vi "CreateCommands.vi"   [LabVIEW 2011]
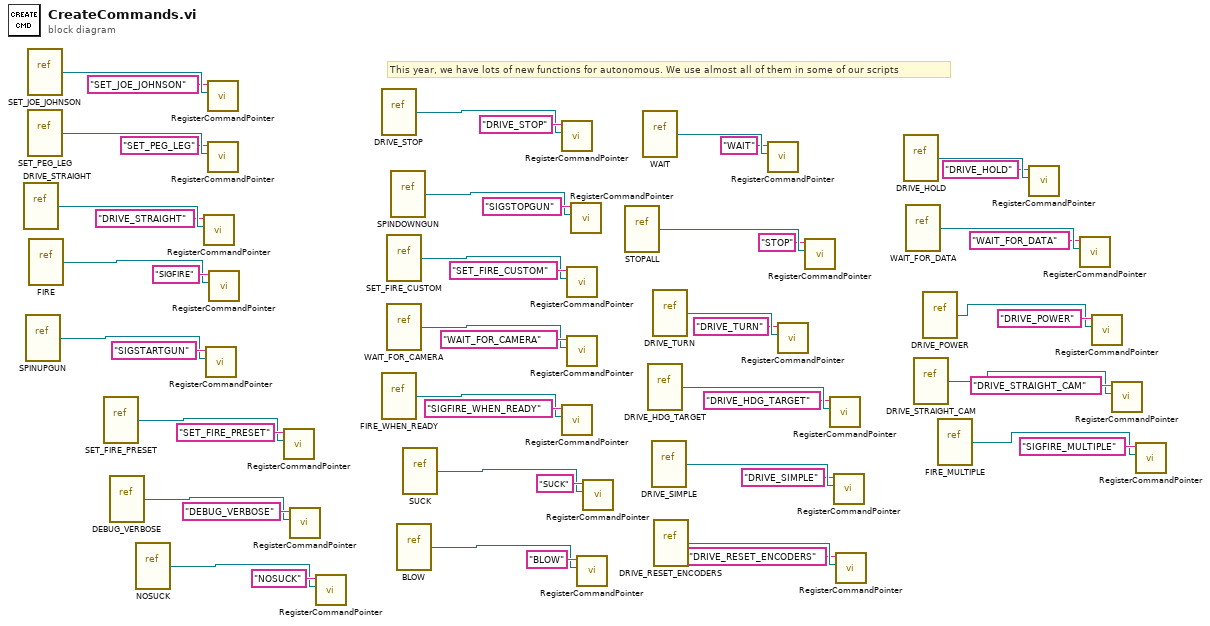
[diagram p0: block diagram]
diagram:
  # "This year, we have lots of new functions for autonomous. We use almost all of them in some of our scripts"
  n1 = vi-ref "DRIVE_STRAIGHT.vi"() -> (w44:refnum<vi>)
  n2 = vi-ref "SPINUPGUN.vi"() -> (w39:refnum<vi>)
  n3 = vi-ref "SET_JOE_JOHNSON.vi"() -> (w48:refnum<vi>)
  n4 = vi-ref "SET_PEG_LEG.vi"() -> (w46:refnum<vi>)
  n5 = vi-ref "FIRE.vi"() -> (w41:refnum<vi>)
  n6 = vi-ref "SET_FIRE_PRESET.vi"() -> (w37:refnum<vi>)
  n7 = vi-ref "DEBUG_VERBOSE.vi"() -> (w35:refnum<vi>)
  n8 = vi-ref "NOSUCK.vi"() -> (w33:refnum<vi>)
  n9 = call "RegisterCommandPointer.vi"("Strict-Typed VI Refnum"=w44, "Name"="DRIVE_STRAIGHT") -> ()  [unwired: 10 out]
  n10 = call "RegisterCommandPointer.vi"("Strict-Typed VI Refnum"=w39, "Name"="SIGSTARTGUN") -> ()  [unwired: 10 out]
  n11 = call "RegisterCommandPointer.vi"("Strict-Typed VI Refnum"=w48, "Name"="SET_JOE_JOHNSON") -> ()  [unwired: 10 out]
  n12 = call "RegisterCommandPointer.vi"("Strict-Typed VI Refnum"=w46, "Name"="SET_PEG_LEG") -> ()  [unwired: 10 out]
  n13 = call "RegisterCommandPointer.vi"("Strict-Typed VI Refnum"=w41, "Name"="SIGFIRE") -> ()  [unwired: 10 out]
  n14 = call "RegisterCommandPointer.vi"("Strict-Typed VI Refnum"=w37, "Name"="SET_FIRE_PRESET") -> ()  [unwired: 10 out]
  n15 = call "RegisterCommandPointer.vi"("Strict-Typed VI Refnum"=w35, "Name"="DEBUG_VERBOSE") -> ()  [unwired: 10 out]
  n16 = call "RegisterCommandPointer.vi"("Strict-Typed VI Refnum"=w33, "Name"="NOSUCK") -> ()  [unwired: 10 out]
  n17 = vi-ref "DRIVE_STOP.vi"() -> (w19:refnum<vi>)
  n18 = vi-ref "FIRE_WHEN_READY.vi"() -> (w27:refnum<vi>)
  n19 = vi-ref "SET_FIRE_CUSTOM.vi"() -> (w23:refnum<vi>)
  n20 = vi-ref "WAIT_FOR_CAMERA.vi"() -> (w25:refnum<vi>)
  n21 = vi-ref "SPINDOWNGUN.vi"() -> (w21:refnum<vi>)
  n22 = vi-ref "BLOW.vi"() -> (w31:refnum<vi>)
  n23 = vi-ref "SUCK.vi"() -> (w29:refnum<vi>)
  n24 = call "RegisterCommandPointer.vi"("Strict-Typed VI Refnum"=w19, "Name"="DRIVE_STOP") -> ()  [unwired: 10 out]
  n25 = call "RegisterCommandPointer.vi"("Strict-Typed VI Refnum"=w27, "Name"="SIGFIRE_WHEN_READY") -> ()  [unwired: 10 out]
  n26 = call "RegisterCommandPointer.vi"("Strict-Typed VI Refnum"=w23, "Name"="SET_FIRE_CUSTOM") -> ()  [unwired: 10 out]
  n27 = call "RegisterCommandPointer.vi"("Strict-Typed VI Refnum"=w25, "Name"="WAIT_FOR_CAMERA") -> ()  [unwired: 10 out]
  n28 = call "RegisterCommandPointer.vi"("Strict-Typed VI Refnum"=w21, "Name"="SIGSTOPGUN") -> ()  [unwired: 10 out]
  n29 = call "RegisterCommandPointer.vi"("Strict-Typed VI Refnum"=w31, "Name"="BLOW") -> ()  [unwired: 10 out]
  n30 = call "RegisterCommandPointer.vi"("Strict-Typed VI Refnum"=w29, "Name"="SUCK") -> ()  [unwired: 10 out]
  n31 = vi-ref "STOPALL.vi"() -> (w52:refnum<vi>)
  n32 = vi-ref "WAIT.vi"() -> (w50:refnum<vi>)
  n33 = vi-ref "DRIVE_HDG_TARGET.vi"() -> (w16:refnum<vi>)
  n34 = vi-ref "DRIVE_SIMPLE.vi"() -> (w14:refnum<vi>)
  n35 = vi-ref "DRIVE_TURN.vi"() -> (w18:refnum<vi>)
  n36 = vi-ref "DRIVE_RESET_ENCODERS.vi"() -> (w12:refnum<vi>)
  n37 = call "RegisterCommandPointer.vi"("Strict-Typed VI Refnum"=w50, "Name"="WAIT") -> ()  [unwired: 10 out]
  n38 = call "RegisterCommandPointer.vi"("Strict-Typed VI Refnum"=w18, "Name"="DRIVE_TURN") -> ()  [unwired: 10 out]
  n39 = call "RegisterCommandPointer.vi"("Strict-Typed VI Refnum"=w52, "Name"="STOP") -> ()  [unwired: 10 out]
  n40 = call "RegisterCommandPointer.vi"("Strict-Typed VI Refnum"=w16, "Name"="DRIVE_HDG_TARGET") -> ()  [unwired: 10 out]
  n41 = call "RegisterCommandPointer.vi"("Strict-Typed VI Refnum"=w14, "Name"="DRIVE_SIMPLE") -> ()  [unwired: 10 out]
  n42 = call "RegisterCommandPointer.vi"("Strict-Typed VI Refnum"=w12, "Name"="DRIVE_RESET_ENCODERS") -> ()  [unwired: 10 out]
  n43 = vi-ref "DRIVE_HOLD.vi"() -> (w10:refnum<vi>)
  n44 = vi-ref "WAIT_FOR_DATA.vi"() -> (w8:refnum<vi>)
  n45 = vi-ref "DRIVE_STRAIGHT_CAM.vi"() -> (w3:refnum<vi>)
  n46 = vi-ref "DRIVE_POWER.vi"() -> (w5:refnum<vi>)
  n47 = vi-ref "FIRE_MULTIPLE.vi"() -> (w1:refnum<vi>)
  n48 = call "RegisterCommandPointer.vi"("Strict-Typed VI Refnum"=w10, "Name"="DRIVE_HOLD") -> ()  [unwired: 10 out]
  n49 = call "RegisterCommandPointer.vi"("Strict-Typed VI Refnum"=w8, "Name"="WAIT_FOR_DATA") -> ()  [unwired: 10 out]
  n50 = call "RegisterCommandPointer.vi"("Strict-Typed VI Refnum"=w5, "Name"="DRIVE_POWER") -> ()  [unwired: 10 out]
  n51 = call "RegisterCommandPointer.vi"("Strict-Typed VI Refnum"=w3, "Name"="DRIVE_STRAIGHT_CAM") -> ()  [unwired: 10 out]
  n52 = call "RegisterCommandPointer.vi"("Strict-Typed VI Refnum"=w1, "Name"="SIGFIRE_MULTIPLE") -> ()  [unwired: 10 out]
